vi "Convert Decimal to SNAFU.vi"(11 "Decimal":i64) -> (3 "SNAFU Number":T1)   [LabVIEW 2020]
uses:
  Cluster SNAFU Number.ctl
  ENUM_SNAFU Digit.ctl
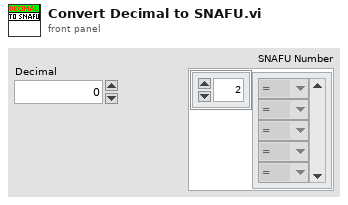
[diagram p1: front panel]
types:
  T1 = typedef "Cluster SNAFU Number.ctl" = cluster{"Digits":T2[]}
  T2 = typedef "ENUM_SNAFU Digit.ctl" = enum16{"=", "-", "0", "1", "2"}
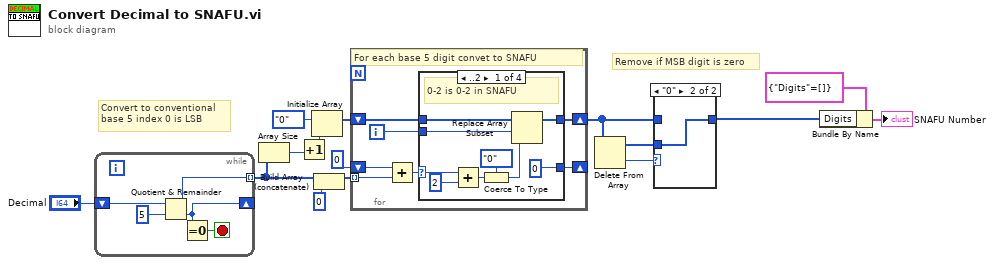
[diagram p0: block diagram]
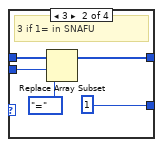
[diagram p3: hidden frame]
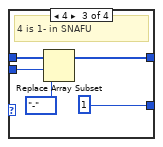
[diagram p4: hidden frame]
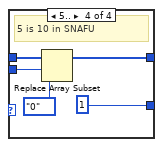
[diagram p5: hidden frame]
diagram:
  # "Convert to conventional\nbase 5 index 0 is LSB"
  # "Remove if MSB digit is zero"
  n1 = while {
    shift-right: [w17] -> _
    shift-left: "Decimal" -> [w20]
    tunnel: [w18] -> w14 mode=indexing
    stop <- w16 stop-if-true
    n2 = Quotient & Remainder(x=w20, y=i64 5) -> (x-y*floor(x/y)=w18:i64, floor(x/y)=w17:i64)
    n3 = Equal To 0?(x=w17) -> (x = 0?=w16:bool)
  }
  n4 = Array Size(array=w14) -> (size(s)=w13:i32)
  n5 = Increment(x=w13) -> (x+1=w12:i32)
  n6 = Initialize Array(ENUM_SNAFU_Digit."0" ("SNAFU IDs"), w12) -> (w10:T2[])
  n7 = Build Array (concatenate)(w14, i64 0) -> (w8:i64[])
  n8 = for {
    shift-right: [w26] -> w6
    shift-left: w10 -> [w27]
    tunnel: w8 -> [w22] mode=indexing
    shift-right: [w21] -> _
    shift-left: i64 0 ("y") -> [w24]
    i -> [w25]
    # "For each base 5 digit convet to SNAFU"
    n9 = Add(x=w24, y=w22) -> (x+y=w23:i64)
    n10 = case shown="..2" w23 {
      selector: w23 -> [w30 _ _ _]
      tunnel: w27 -> [w36 w41 w46 w51]
      tunnel: [w35 w40 w45 w50] -> w26
      tunnel: w25 -> [w34 w39 w44 w49]
      tunnel: [i64 0 ("y") i64 1 ("y") i64 1 ("y") i64 1 ("y")] -> w21
      frame ..2 {
        # "0-2 is 0-2 in SNAFU"
        n11 = Add(x=w30, y=i64 2) -> (x+y=w32:i64)
        n12 = Coerce To Type(0:w32, 1:ENUM_SNAFU_Digit."0" ("SNAFU IDs")) -> (2:w29:T2)
        n13 = Replace Array Subset(array=w36, new element=w29, index=w34) -> (w35:T2[])
      }
      frame 3 {
        # "3 if 1= in SNAFU"
        n14 = Replace Array Subset(array=w41, new element=ENUM_SNAFU_Digit."=" ("SNAFU IDs"), index=w39) -> (w40:T2[])
      }
      frame 4 {
        # "4 is 1- in SNAFU"
        n15 = Replace Array Subset(array=w46, new element=ENUM_SNAFU_Digit."-" ("SNAFU IDs"), index=w44) -> (w45:T2[])
      }
      frame 5.. {
        # "5 is 10 in SNAFU"
        n16 = Replace Array Subset(array=w51, new element=ENUM_SNAFU_Digit."0" ("SNAFU IDs"), index=w49) -> (w50:T2[])
      }
    }
  }
  n17 = Delete From Array(array=w6) -> (deleted portion=w5:T2, array with subset deleted=w4:T2[])  [unwired: 2 in]
  n18 = case shown="\"0\"" w5 {
    tunnel: w6 -> [w52 _]
    tunnel: w4 -> [_ w53]
    tunnel: [w52 w53] -> w2
    frame Default {
    }
    frame "0" {
    }
  }
  n19 = Bundle By Name(cluster=T1 {"Digits"=[]} ("SNAFU NUMBER"), "Digits"=w2) -> (→"SNAFU Number":T1)
